vi "Client Info Loop.vi"(8 "error in (no error)":errorcluster, 11 "TCPMessaging in":refnum<class "TCPMessaging.lvclass">) -> (0 "error out":errorcluster)   [LabVIEW 2020, in "Vecto.lvlib" / "TCPMessaging.lvclass"]
doc: "Maintains the list of currently connected clients."
uses:
  TCPMessaging.lvclass
  TCPMessaging.lvclass/TCPMessaging.ctl
  proto/TcpClientHello/Data.ctl
  proto/TcpClientHello/TcpClientHello.lvlib
  Client Info.ctl
  Vecto.lvlib
  Client Info Loop Data.ctl
  Connected Client.ctl
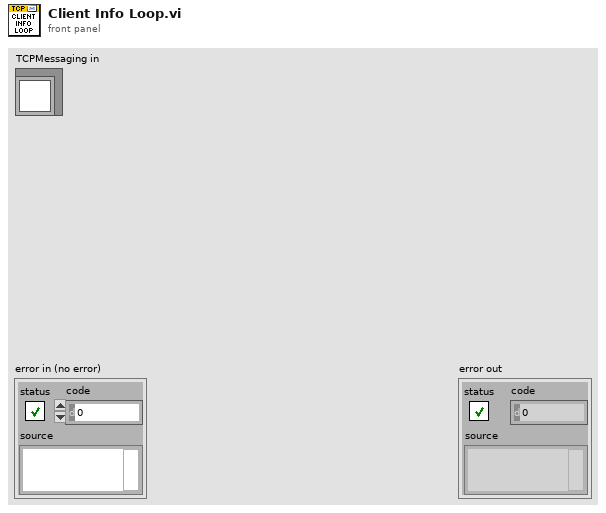
[diagram p1: front panel]
types:
  T1 = typedef "Vecto.lvlib/TCPMessaging.lvclass/Client Info Loop Data.ctl" = cluster{"Map":map{string, T2}}
  T2 = typedef "Vecto.lvlib/TCPMessaging.lvclass/Connected Client.ctl" = cluster{"TCP":refnum<k5>, "Client Info":T3, "TX Q":refnum<queue>}
  T3 = typedef "Vecto.lvlib/Client Info.ctl" = cluster{"TcpClientHello":T4, "Remote Address":string, "Remote Port":u16}
  T4 = typedef "TcpClientHello.lvlib/Data.ctl" = cluster{"node_id":u32, "system":string, "cluster":string, "node_name":string, "app_version":string, "config_version":string}
  T5 = typedef "Vecto.lvlib/TCPMessaging.lvclass/Client Action Data.ctl" = cluster{"Client Action":T6, "Client Info":T3, "TCP":refnum<k5>, "TX Q":refnum<queue>}
  T6 = typedef "Vecto.lvlib/TCPMessaging.lvclass/Client Action.ctl" = enum16{"Connect", "Ready", "Disconnect"}
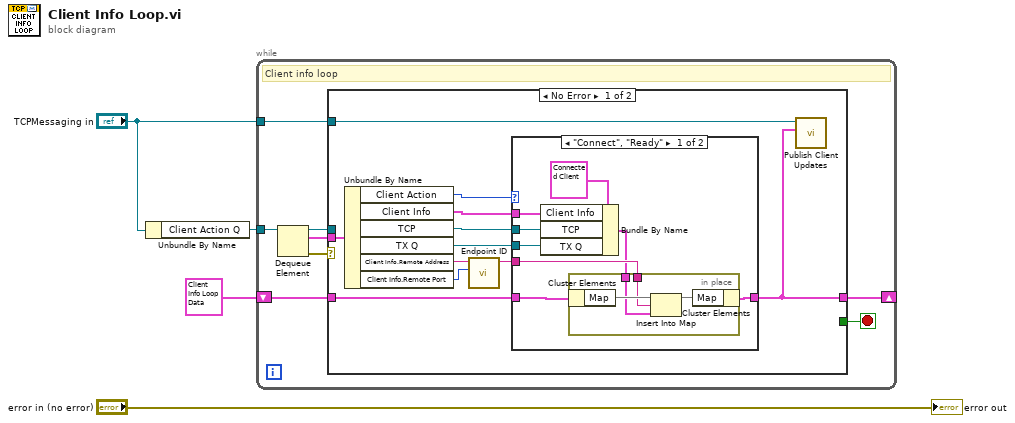
[diagram p0: block diagram]
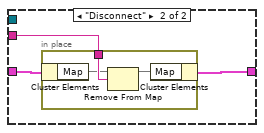
[diagram p2: hidden frame]
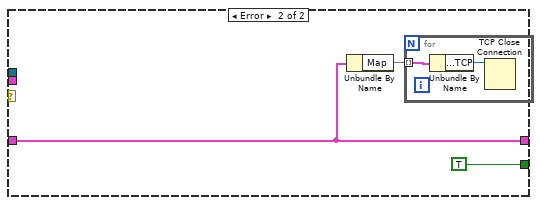
[diagram p3: hidden frame]
diagram:
  n1 = Unbundle By Name("TCPMessaging in") -> ("Client Action Q"=w2:refnum<queue>)
  n2 = while {
    tunnel: w2 -> [w12]
    shift-right: [w8] -> _
    shift-left: T1 {"Map"={}} ("Client Info Loop Data") -> [w9]
    tunnel: "TCPMessaging in" -> [w5]
    stop <- w7 stop-if-true
    # "Client info loop"
    n3 = Dequeue Element(queue=w12) -> (queue out=w6:refnum<queue>, element=w10:T5, error out=w11:errorcluster)  [unwired: 2 in, 1 out]
    n4 = case shown="No Error" w11 {
      tunnel: w10 -> [w23 _]
      tunnel: w9 -> [w18 w43]
      tunnel: [w13 w43] -> w8
      tunnel: [_ TRUE] -> w7
      tunnel: w6 -> [_ _]
      tunnel: w5 -> [w14 _]
      frame No Error {
        n5 = Unbundle By Name(w23) -> ("Client Action"=w20:T6, "Client Info"=w17:T3, "TCP"=w16:refnum<k5>, "TX Q"=w15:refnum<queue>, "Client Info.Remote Address"=w22:string, "Client Info.Remote Port"=w21:u16)
        n6 = call "Endpoint ID.vi"("Remote Port"=w21, "Remote Address"=w22) -> ("Endpoint ID"=w19:string)  [unwired: 9 in]
        n7 = case shown="\"Connect\", \"Ready\"" w20 {
          tunnel: w19 -> [w29 w36]
          tunnel: w18 -> [w31 w38]
          tunnel: [w30 w37] -> w13
          tunnel: w17 -> [w26 _]
          tunnel: w16 -> [w25 _]
          tunnel: w15 -> [w24 _]
          frame "Connect", "Ready" {
            n8 = Bundle By Name(cluster=T2 {"TCP"=refnum, "Client Info"={"TcpClientHello"={"node_id"=0, "system"="", "cluster"="", "node_name"="", "app_version"="", "config_version"=""}, "Remote Address"="", "Remote Port"=0}, "TX Q"=refnum} ("Connected Clients"), "Client Info"=w26, "TCP"=w25, "TX Q"=w24) -> (w27:T2)
            n9 = in-place {
              in-place-border: w29 -> [w34]
              in-place-border: w27 -> [w33]
              n10 = in-place-cluster #1(w31) -> ("Map"=w35:map{string, T2})
              n11 = Insert Into Map(map in=w35, key=w34, value=w33) -> (map out=w32:map{string, T2})  [unwired: 2 out]
              n12 = in-place-cluster #1("Map"=w32) -> (w30:T1)
            }
          }
          frame "Disconnect" {
            n13 = in-place {
              in-place-border: w36 -> [w41]
              n14 = in-place-cluster #2(w38) -> ("Map"=w40:map{string, T2})
              n15 = Remove From Map(10:w41, 11:w40) -> (3:w39:map{string, T2})  [unwired: 2 out]
              n16 = in-place-cluster #2("Map"=w39) -> (w37:T1)
            }
          }
        }
        n17 = call "Publish Client Updates.vi"("Client Info Loop Data"=w13, "TCPMessaging in"=w14) -> ()  [unwired: 8 in, 2 out]
      }
      frame Error {
        n18 = Unbundle By Name(w43) -> ("Map"=w42:map{string, T2})
        n19 = for {
          tunnel: w42 -> [w46] mode=indexing
          n20 = Unbundle By Name(w46) -> ("Connected Client.TCP"=w45:refnum<k5>)
          n21 = TCP Close Connection(connection ID=w45) -> ()  [unwired: 2 in, 2 out]
        }
      }
    }
  }
  "error out" <- "error in (no error)"
